vi "CRIO_TCPStateSelector.vi"(8 "error in (no error)":errorcluster, 10 "Curr State":T1, 11 "data in":string) -> (0 "error out":errorcluster, 3 "Command State":T1)   [LabVIEW 2017]
uses:
  CRIO_StateEnum.ctl
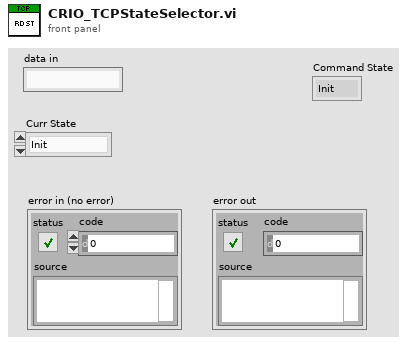
[diagram p1: front panel]
types:
  T1 = typedef "CRIO_StateEnum.ctl" = enum16{"Init", "Listen", "Wait", "Setup", "Ready to Launch", "Start Flight", "Accelerating", "Coasting", "Braking", "End Flight", "Loading", "Stop"}
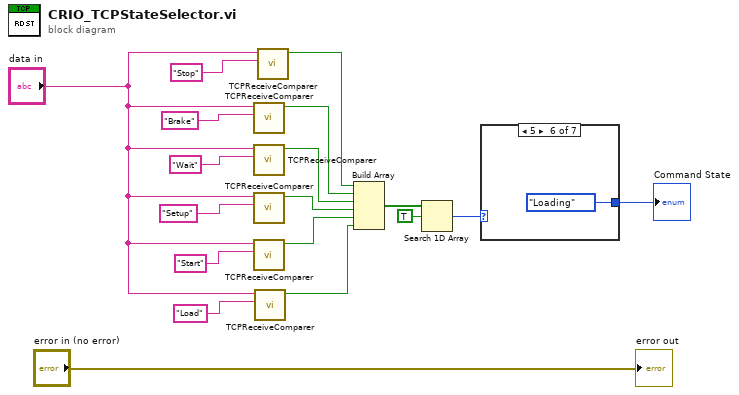
[diagram p0: block diagram]
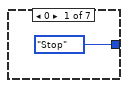
[diagram p2: hidden frame]
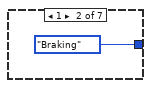
[diagram p3: hidden frame]
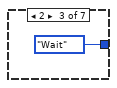
[diagram p4: hidden frame]
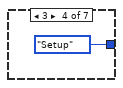
[diagram p5: hidden frame]
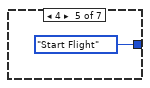
[diagram p6: hidden frame]
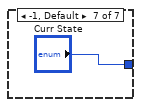
[diagram p7: hidden frame]
diagram:
  n1 = call "TCPReceiveComparer.vi"("Compare String"="Brake" ("y"), "Recieved String"="data in") -> ("Match"=w16:bool)  [unwired: 9 in]
  n2 = call "TCPReceiveComparer.vi"("Compare String"="Wait" ("y"), "Recieved String"="data in") -> ("Match"=w12:bool)  [unwired: 9 in]
  n3 = call "TCPReceiveComparer.vi"("Compare String"="Setup" ("y"), "Recieved String"="data in") -> ("Match"=w11:bool)  [unwired: 9 in]
  n4 = call "TCPReceiveComparer.vi"("Compare String"="Start" ("y"), "Recieved String"="data in") -> ("Match"=w10:bool)  [unwired: 9 in]
  n5 = call "TCPReceiveComparer.vi"("Compare String"="Load" ("y"), "Recieved String"="data in") -> ("Match"=w1:bool)  [unwired: 9 in]
  n6 = call "TCPReceiveComparer.vi"("Compare String"="Stop" ("y"), "Recieved String"="data in") -> ("Match"=w4:bool)  [unwired: 9 in]
  n7 = Build Array(w4, w16, w12, w11, w10, w1) -> (w8:bool[])
  n8 = Search 1D Array(1D array=w8, element=TRUE) -> (index of element=w7:i32)  [unwired: 1 in]
  n9 = case shown="5" w7 {
    tunnel: [CRIO_StateEnum."Stop" ("States") CRIO_StateEnum."Braking" ("States") CRIO_StateEnum."Wait" ("States") CRIO_StateEnum."Setup" ("States") CRIO_StateEnum."Start Flight" ("States") CRIO_StateEnum."Loading" ("States") "Curr State"] -> w6
    frame 0 {
    }
    frame 1 {
    }
    frame 2 {
    }
    frame 3 {
    }
    frame 4 {
    }
    frame 5 {
    }
    frame -1, Default {
    }
  }
  "Command State" <- w6
  "error out" <- "error in (no error)"
